vi "memory to strings.vi"(8 "error in":errorcluster, 11 "memory hierarchy":T4) -> (0 "error out":errorcluster, 3 "1.0.0":T1)   [LabVIEW 2013, in "NISE_CEF_TreeSerializer.lvlib"]
uses:
  NISE_CEF_TreeSerializer.lvlib
  memory hierarchy.ctl
  hierarchy element.ctl
  serializable configuration/NISE_CEF_serializable configuration.lvclass
  file data format.ctl
  instance data.ctl
  serializable configuration/NISE_CEF_serializable configuration.lvclass/NISE_CEF_serializable configuration.ctl
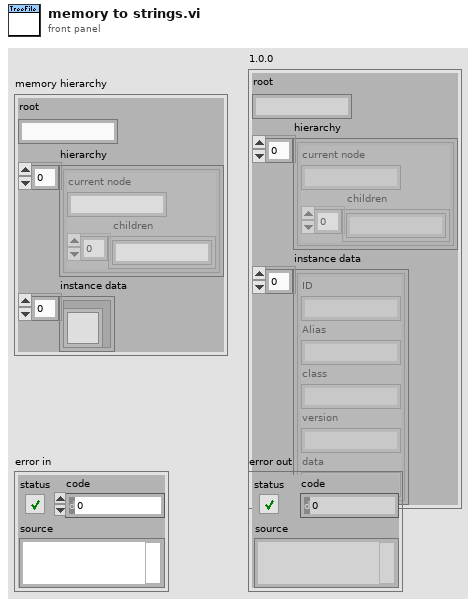
[diagram p1: front panel]
types:
  T1 = typedef "NISE_CEF_TreeSerializer.lvlib/file data format.ctl" = cluster{"root":string, "hierarchy":T2[], "instance data":T3[]}
  T2 = typedef "NISE_CEF_TreeSerializer.lvlib/hierarchy element.ctl" = cluster{"current node":string, "children":string[]}
  T3 = typedef "NISE_CEF_TreeSerializer.lvlib/instance data.ctl" = cluster{"ID":string, "Alias":string, "class":string, "version":string, "data":string}
  T4 = typedef "NISE_CEF_TreeSerializer.lvlib/memory hierarchy.ctl" = cluster{"root":string, "hierarchy":T2[], "instance data":refnum<class "NISE_CEF_serializable configuration.lvclass">[]}
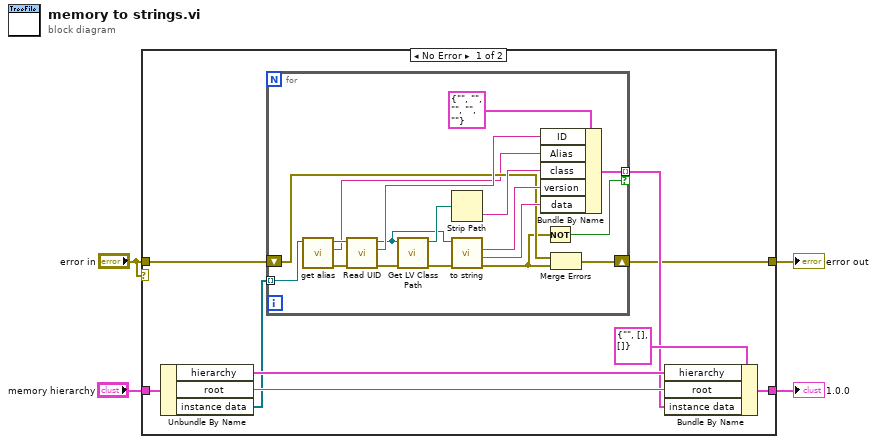
[diagram p0: block diagram]
diagram:
  n1 = case shown="No Error" "error in" {
    tunnel: "memory hierarchy" -> [w13 _]
    tunnel: [w11 _] -> w3
    tunnel: [w6 w32] -> w2
    tunnel: "error in" -> [w5 w32]
    frame No Error {
      n2 = Unbundle By Name(w13) -> ("hierarchy"=w10:T2[], "root"=w9:string, "instance data"=w7:refnum<class "NISE_CEF_serializable configuration.lvclass">[])
      n3 = for {
        tunnel: [w30] -> w8 mode=indexing if=w20
        tunnel: w7 -> [w16] mode=indexing
        shift-right: [w17] -> w6
        shift-left: w5 -> [w19]
        n4 = call "get alias.vi"("configuration in"=w16) -> ("error out"=w21:errorcluster, "alias"=w14:string, "configuration out"=w15:refnum<class "NISE_CEF_serializable configuration.lvclass">)  [unwired: 8 in]
        n5 = call "Read UID.vi"("error in"=w21, "configuration in"=w15) -> ("error out"=w22:errorcluster, "instance id"=w27:string, "configuration out"=w24:refnum<class "NISE_CEF_serializable configuration.lvclass">)  [unwired: 7 in]
        n6 = call <vilib>:"Get LV Class Path.vi"("error in (no error)"=w22, "object"=w24) -> ("error out"=w23:errorcluster, "class path"=w29:path)  [unwired: 8 in]
        n7 = Strip Path(path=w29) -> (name=w28:string)  [unwired: 1 out]
        n8 = call-dynamic "to string.vi"("error in"=w23, "configuration in"=w24) -> ("error out"=w18:errorcluster, "data"=w25:string, "version"=w26:string)  [unwired: 6 in, 1 out]
        n9 = Bundle By Name(cluster=T3 {"ID"="", "Alias"="", "class"="", "version"="", "data"=""} ("instancedata"), "ID"=w27, "Alias"=w14, "class"=w28, "version"=w26, "data"=w25) -> (w30:T3)
        n10 = Not(x=w18) -> (.not. x?=w20:bool)
        n11 = Merge Errors(w19, w18) -> (w17:errorcluster)
      }
      n12 = Bundle By Name(cluster=T1 {"root"="", "hierarchy"=[], "instance data"=[]} ("1.0.0"), "hierarchy"=w10, "root"=w9, "instance data"=w8) -> (w11:T1)
    }
    frame Error {
    }
  }
  "1.0.0" <- w3
  "error out" <- w2
